vi "Send Steps with Request Server ID.vi"(8 "error in (no error)":errorcluster, 9 "Write Data?":bool=TRUE, 10 "Command.Steps":i32, 11 "Model in":refnum<class "Model.lvclass">) -> (0 "error out":errorcluster, 3 "Model out":refnum<class "Model.lvclass">)   [LabVIEW 2016, in "Model.lvclass"]
uses:
  Model.lvclass
  <vilib>/Platform/TimedLoop/XDataNode/timing_clust.ctl
  <vilib>/Platform/TimedLoop/XDataNode/nitl_modes.ctl
  <vilib>/Platform/TimedLoop/XDataNode/wakeup.ctl
  Model.lvclass/Model.ctl
  common_rt_hpilc/HPILC/HPILC.lvclass/HPILC.ctl
  common_rt_hpilc/HPILC/HPILC.lvclass
  C:/CODE/ts_hpmt/common_rt_ilc/ILC/ILC.lvclass
  <vilib>/platform/TimedLoop/XDataNode/XDataNode.xnode
  Modbus/DesktopModbus/DesktopModbus.lvclass
  <vilib>/Platform/TimedLoop/XDataNode/XDNodeRunTimeDep.lvlib
  common_rt_ilc/ILC/ILC.lvclass
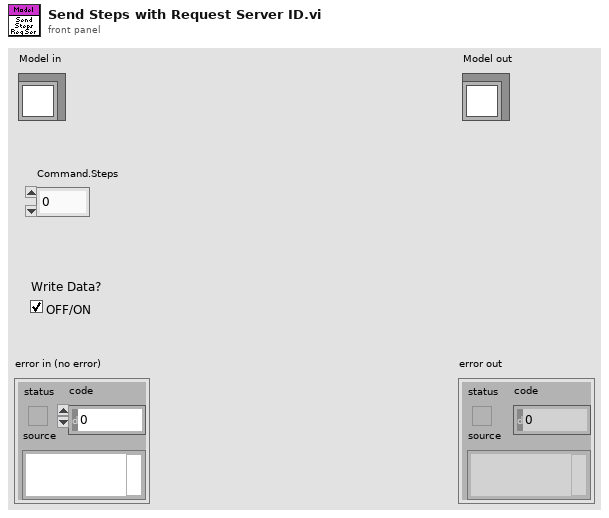
[diagram p1: front panel]
types:
  T1 = typedef "XDNodeRunTimeDep.lvlib/timing_clust.ctl" = cluster{"Expected End [f-1]":u64, "Actual End [f-1]":u64, "Finished Late? [f-1]":bool, "Expected End [i-1]":u64, "Actual End [i-1]":u64, "Finished Late? [i-1]":bool, "Expected Start [i]":u64, "Actual Start [i]":u64, "Expected Start [f]":u64, "Actual Start [f]":u64, "Source Name":string, "Structure Name":string, "Period":i64, "Deadline":i64, "Offset":i64, "Start":i64, "Priority":i32, "Timeout":i32, "Mode":T2, "Wakeup Reason":T3, "Error":errorcluster, "Source Type":string, "Secondary Source Type":string, "Global End Time":u64, "Global Start Time":u64, "Frame Duration":u64, "Iteration Duration":u64, "Assigned CPU":i32, "I/O Scan Engine Mode":u32}
  T2 = typedef "XDNodeRunTimeDep.lvlib/nitl_modes.ctl" = enum32{"No Change", "Process missed periods, maintain original phase", "Discard missed periods, maintain original phase", "Process missed periods, ignore original phase", "Discard missed periods, ignore original phase"}
  T3 = typedef "XDNodeRunTimeDep.lvlib/wakeup.ctl" = enum32{"Normal", "Aborted", "Asynchronous wakeup", "Timing source error", "Timed loop error", "Timeout"}
  T4 = typedef "RTHPILC.lvlib/HPData.ctl" = cluster{"Constants":T5, "Command":T6, "Telemetry":T7, "Responses":T8, "Timings":T10}
  T5 = typedef "RTHPILC.lvlib/HPConstants.ctl" = cluster{"ID":i16, "ReferencePosition":i32}
  T6 = typedef "RTHPILC.lvlib/HPCommand.ctl" = cluster{"Steps":i8}
  T7 = typedef "RTHPILC.lvlib/HPTelemetry.ctl" = cluster{"ILCFault":bool, "LimitSwitchCWOperated":bool, "LimitSwitchCCWOperated":bool, "BroadcastCounter":u8, "SSIEncoderValue":i32, "LoadCellForce":sgl}
  T8 = typedef "RTHPILC.lvlib/HPResponses.ctl" = cluster{"StepMotor":T9, "ForceAndStatus":T9}
  T9 = typedef "RTModbus.lvlib/ExceptionCodes.ctl" = u16
  T10 = typedef "RTHPILC.lvlib/HPTimings.ctl" = cluster{"BroadcastStepMotor":u32, "ForceAndStatus":u32, "FreezeSensorValues":u32, "StepMotor":u32}
  T11 = typedef "RTModbus.lvlib/TxFrame.ctl" = cluster{"Data":u8[], "WaitForTrigger":bool, "WaitForRx":u16, "TriggerIRQ":bool, "DelayMicroseconds":u16, "DelayMilliseconds":u16, "Timestamp":bool}
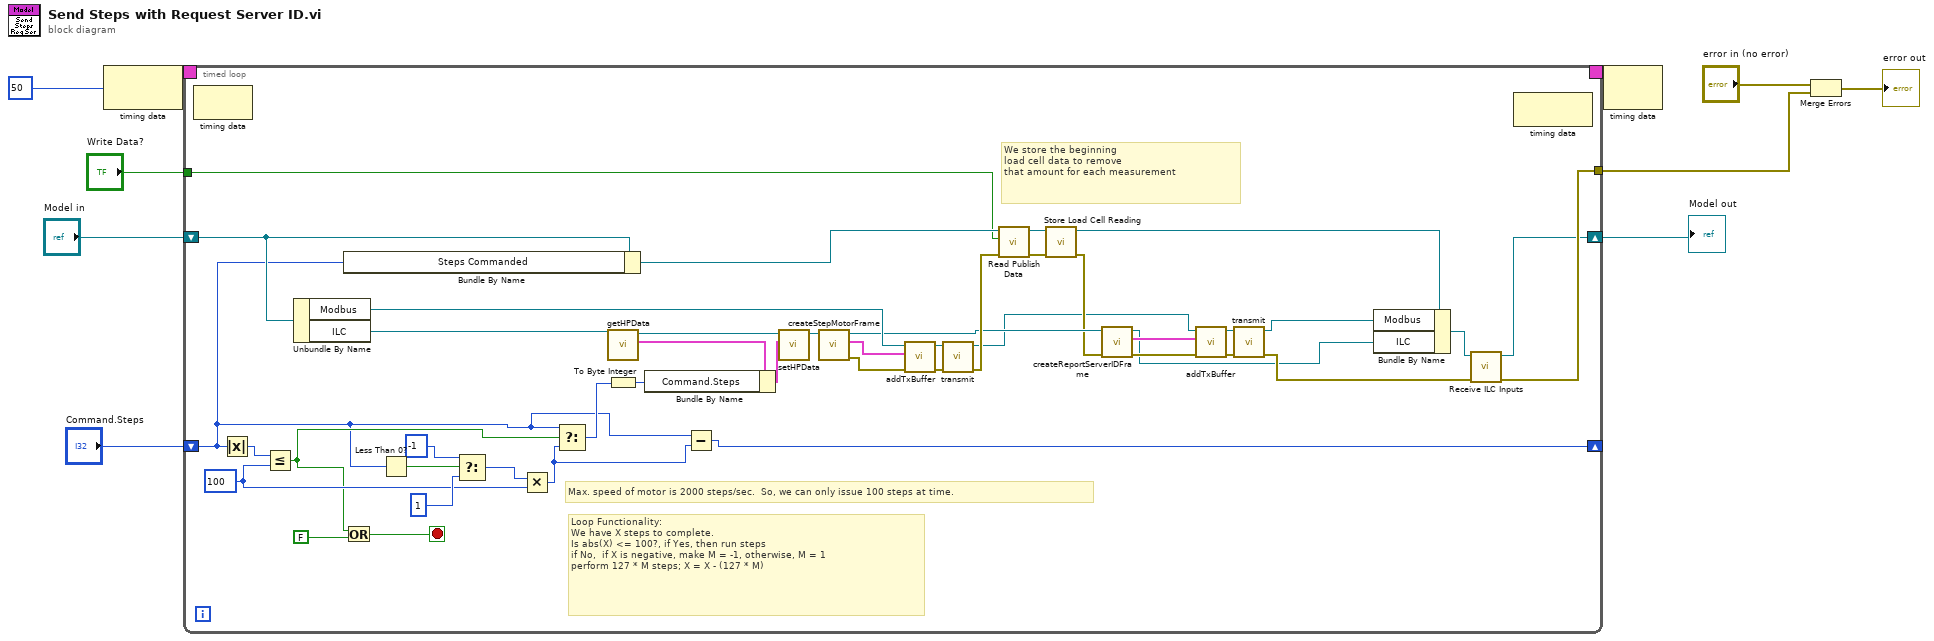
[diagram p0: block diagram]
diagram:
  n1 = node-c288(i64 50 ("Period")) -> (w6:T1)
  n2 = timed-loop {
    shift-right: [w37] -> _
    shift-left: "Command.Steps" -> [w28]
    shift-right: [w11] -> w3
    shift-left: "Model in" -> [w29]
    timing: w6 -> [_]
    timing-out: [_] -> w5
    tunnel: "Write Data?" -> [w25]
    tunnel: [w15] -> w1
    stop <- w43 stop-if-true
    w40 = 100
    # "We store the beginning\nload cell data to remove\nthat amount for each measurement"
    # "Loop Functionality:\nWe have X steps to complete. \nIs abs(X) <= 100?, if Yes, then run steps\nif No,  if X is negative, make M = -1, otherwise, M = 1\nperform 127 * M steps; X = X - (127 * M)"
    # "Max. speed of motor is 2000 steps/sec.  So, we can only issue 100 steps at time."
    n3 = node-c288() -> ()  [unwired: 1 in, 1 out]
    n4 = Absolute Value(x=w28) -> (abs(x)=w46:i32)
    n5 = Less Or Equal?(x=w46, y=w40) -> (x <= y?=w36:bool)
    n6 = Unbundle By Name(w29) -> ("Modbus"=w32:refnum<class "DesktopModbus.lvclass">, "ILC"=w31:refnum<class "HPILC.lvclass">)
    n7 = Bundle By Name(cluster=w29, "Steps Commanded"=w28) -> (w27:refnum<class "Model.lvclass">)
    n8 = Or(x=w36, y=FALSE) -> (x .or. y?=w43:bool)
    n9 = Less Than 0?(x=w28) -> (x < 0?=w35:bool)
    n10 = Select(t=-1, s=w35, f=1) -> (s? t:f=w41:i32)
    n11 = Multiply(x=w41, y=w40) -> (x*y=w38:i32)
    n12 = Select(t=w28, s=w36, f=w38) -> (s? t:f=w33:i32)
    n13 = call "getHPData.vi"("HPILC in"=w31) -> ("HPData"=w54:T4, "HPILC out"=w53:refnum<class "HPILC.lvclass">)  [unwired: 9 in]
    n14 = To Byte Integer(number=w33) -> (8bit integer=w39:i8)
    n15 = Bundle By Name(cluster=w54, "Command.Steps"=w39) -> (w47:T4)
    n16 = Subtract(x=w28, y=w38) -> (x-y=w37:i32)
    n17 = call "setHPData.vi"("HPData"=w47, "HPILC in"=w53) -> ("HPILC out"=w52:refnum<class "HPILC.lvclass">)  [unwired: 9 in]
    n18 = call "createStepMotorFrame.vi"("HPILC in"=w52) -> ("error out"=w49:errorcluster, "TxFrame"=w50:T11, "HPILC out"=w24:refnum<class "HPILC.lvclass">)  [unwired: 8 in]
    n19 = call-dynamic "addTxBuffer.vi"("error in (no error)"=w49, "TxFrame"=w50, "DesktopModbus in"=w32) -> ("error out"=w48:errorcluster, "DesktopModbus out"=w51:refnum<class "DesktopModbus.lvclass">)  [unwired: 7 in]
    n20 = call-dynamic "transmit.vi"("error in (no error)"=w48, "DesktopModbus in"=w51) -> ("error out"=w34:errorcluster, "DesktopModbus out"=w21:refnum<class "DesktopModbus.lvclass">)  [unwired: 8 in]
    n21 = call "Read Publish Data.vi"("error in (no error)"=w34, "Write Data?"=w25, "Model in"=w27) -> ("error out"=w26:errorcluster, "Model out"=w30:refnum<class "Model.lvclass">)  [unwired: 7 in]
    n22 = call "Store Load Cell Reading.vi"("error in (no error)"=w26, "Model in"=w30) -> ("error out"=w23:errorcluster, "Model out"=w13:refnum<class "Model.lvclass">)  [unwired: 8 in]
    n23 = call "createReportServerIDFrame.vi"("error in (no error)"=w23, "ILC in"=w24) -> ("error out"=w18:errorcluster, "TxFrame"=w22:T11, "ILC out"=w14:refnum<class "HPILC.lvclass">)  [unwired: 7 in]
    n24 = call-dynamic "addTxBuffer.vi"("error in (no error)"=w18, "TxFrame"=w22, "DesktopModbus in"=w21) -> ("error out"=w17:errorcluster, "DesktopModbus out"=w20:refnum<class "DesktopModbus.lvclass">)  [unwired: 7 in]
    n25 = call-dynamic "transmit.vi"("error in (no error)"=w17, "DesktopModbus in"=w20) -> ("error out"=w16:errorcluster, "DesktopModbus out"=w19:refnum<class "DesktopModbus.lvclass">)  [unwired: 8 in]
    n26 = Bundle By Name(cluster=w13, "Modbus"=w19, "ILC"=w14) -> (w12:refnum<class "Model.lvclass">)
    n27 = call "Receive ILC Inputs.vi"("error in (no error)"=w16, "Model in"=w12) -> ("error out"=w15:errorcluster, "Model out"=w11:refnum<class "Model.lvclass">)  [unwired: 8 in]
    n28 = node-c288() -> ()  [unwired: 1 in, 1 out]
  }
  "Model out" <- w3
  n29 = node-c288(w5) -> ()  [unwired: 1 out]
  n30 = Merge Errors("error in (no error)", w1) -> (→"error out":errorcluster)
